vi "how to String Count_Concatenantion.vi"() -> ()   [LabVIEW 2020]
panel:
  out "String Length":dbl
  out "Combined String 2":string
  in  "Trailer 2":string
  in  "Numeric":dbl
  in  "Header":string
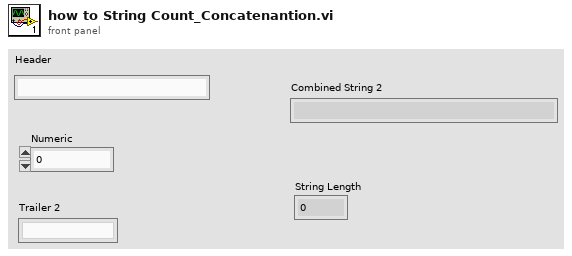
[diagram p1: front panel]
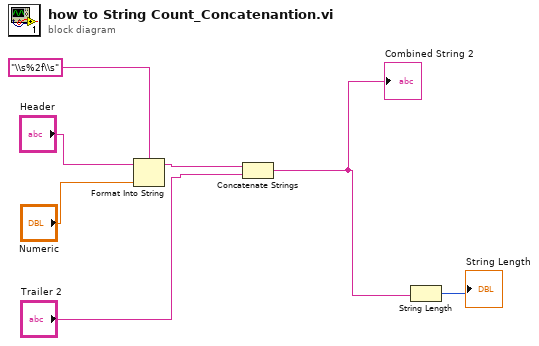
[diagram p0: block diagram]
diagram:
  n1 = Format Into String(format string="\\s%2f\\s", initial string="Header", "Numeric") -> (resulting string=w4:string)  [unwired: 1 in, 1 out]
  n2 = Concatenate Strings(w4, "Trailer 2") -> (w2:string)
  "Combined String 2" <- w2
  n3 = String Length(string=w2) -> (length=→"String Length":i32)
